vi "P3.vi"() -> ()   [LabVIEW 2019]
panel:
  in  "Stop Button":bool
  out "n":dbl
  out "m":dbl
  in  "y2":dbl
  in  "x2":dbl
  in  "y1":dbl
  in  "x1":dbl
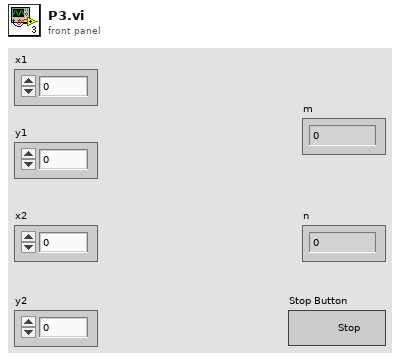
[diagram p1: front panel]
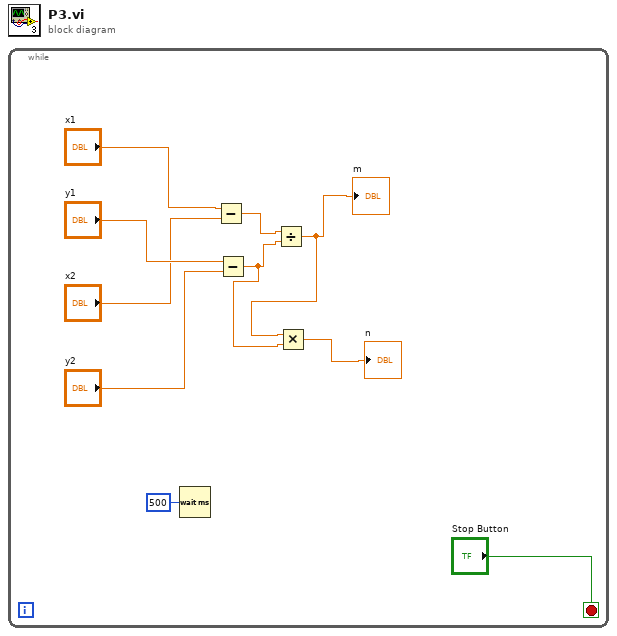
[diagram p0: block diagram]
diagram:
  n1 = while {
    stop <- "Stop Button" stop-if-true
    n2 = Wait (ms)(milliseconds to wait=u32 500) -> ()  [unwired: 1 out]
    n3 = Subtract(x="x1", y="x2") -> (x-y=w6:dbl)
    n4 = Subtract(x="y1", y="y2") -> (x-y=w4:dbl)
    n5 = Divide(x=w6, y=w4) -> (x/y=w5:dbl)
    "m" <- w5
    n6 = Multiply(x=w5, y=w4) -> (x*y=→"n":dbl)
  }
